vi "MotionProfileTest.vi"() -> ()   [LabVIEW 2018]
uses:
  <vilib>/Rock Robotics/WPI/ThirdParty/Phoenix-LabVIEW/Motor Controller/Controls/CTRE_Phoenix_MotorControl_TrajectoryPointTimeDur.ctl
  TypeDefs/MotionProfileGeneratorParams.ctl
panel:
  out "IntegralV":dbl
  out "NumPoints":i32
  out "Update Rate (Hz)":dbl
  in  "stop":bool
  out "Motion Profile":T1(graph)
  in  "Starting Position (units)":dbl
  in  "Acceleration Ramp Time (ms)":dbl=200.0
  in  "Trajectory Point Interval (ms)":T2=10 items=["TrajectoryDuration_0ms"=0, "TrajectoryDuration_5ms"=5, "TrajectoryDuration_10ms"=10, "TrajectoryDuration_20ms"=20, "TrajectoryDuration_30ms"=30, "TrajectoryDuration_40ms"=40, "TrajectoryDuration_50ms"=50, "TrajectoryDuration_100ms"=100]
  in  "Velocity Ramp Time (ms)":dbl=400.0
  in  "Maximum Travel Speed (units/s)":dbl=240.0
  in  "Travel Distance (units)":dbl=5.0
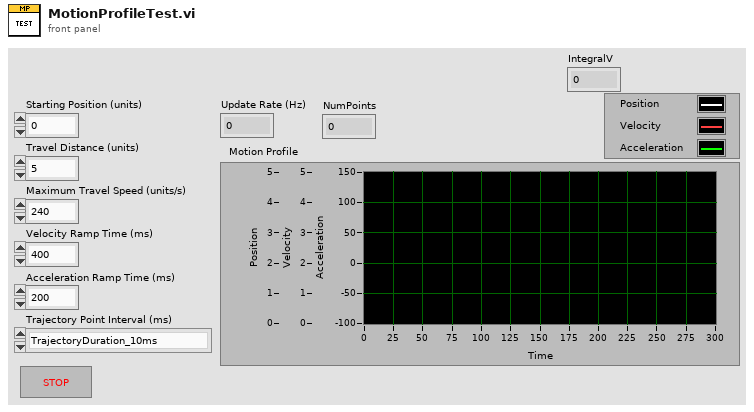
[diagram p1: front panel]
types:
  T1 = cluster{dbl, "Trajectory Point Interval (ms)":i32, dbl[][]}
  T2 = typedef "CTRE_Phoenix_MotorControl_TrajectoryPointTimeDur.ctl" = i32
  T3 = typedef "MotionProfileGeneratorParams.ctl" = cluster{"Trajectory Point Interval (ms)":T2, "Maximum Travel Speed (units/s)":dbl, "Velocity Ramp Time (ms)":dbl, "Acceleration Ramp Time (ms)":dbl}
  T4 = typedef "TrajectoryPoint.ctl" = cluster{"Position ":dbl, "Velocity ":dbl, "Time (ms)":T2, "Last Point":bool}
  T5 = cluster{dbl, "Trajectory Point Interval (ms)":T2, dbl[][]}
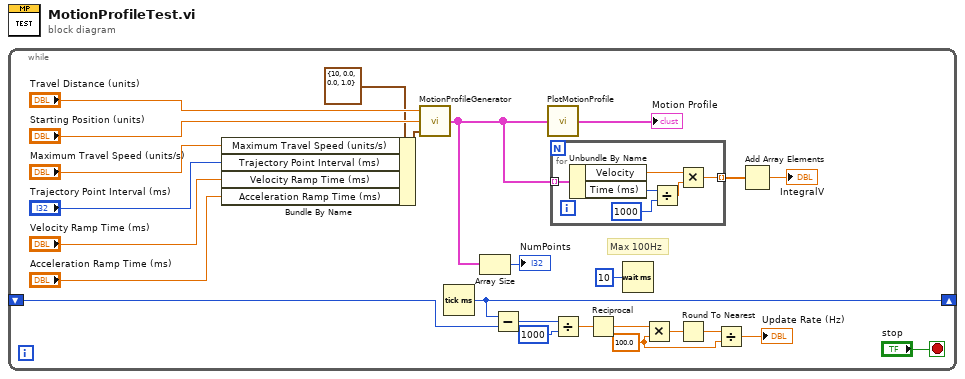
[diagram p0: block diagram]
diagram:
  n1 = while {
    shift-right: [w21] -> _
    shift-left: _ -> [w22]
    stop <- "stop" stop-if-true
    w14 = 100.0 ("y")
    # "Max 100Hz"
    n2 = Bundle By Name(cluster=T3 {"Trajectory Point Interval (ms)"=10, "Maximum Travel Speed (units/s)"=0.0, "Velocity Ramp Time (ms)"=0.0, "Acceleration Ramp Time (ms)"=1.0} ("MotionProfileGeneratorParameters"), "Maximum Travel Speed (units/s)"="Maximum Travel Speed (units/s)", "Trajectory Point Interval (ms)"="Trajectory Point Interval (ms)", "Velocity Ramp Time (ms)"="Velocity Ramp Time (ms)", "Acceleration Ramp Time (ms)"="Acceleration Ramp Time (ms)") -> (w9:T3)
    n3 = call "MotionProfileGenerator.vi"("MotionProfileGeneratorParameters"=w9, "Starting Position (units)"="Starting Position (units)", "Travel Distance (units)"="Travel Distance (units)") -> ("Trajectory Points"=w3:T4[])
    n4 = Tick Count (ms)() -> (millisecond timer value=w21:u32)
    n5 = Array Size(array=w3) -> (size(s)=→"NumPoints":i32)
    n6 = Subtract(x=w21, y=w22) -> (x-y=w20:u32)
    n7 = call "PlotMotionProfile.vi"("Trajectory Points"=w3) -> ("MotionProfileGraph"=→"Motion Profile":T5)
    n8 = for {
      tunnel: w3 -> [w31] mode=indexing
      tunnel: [w29] -> w2 mode=indexing
      n9 = Unbundle By Name(w31) -> ("Velocity"=w30:dbl, "Time (ms)"=w28:T2)
      n10 = Divide(x=w28, y=1000) -> (x/y=w27:dbl)
      n11 = Multiply(x=w30, y=w27) -> (x*y=w29:dbl)
    }
    n12 = Divide(x=w20, y=u32 1000) -> (x/y=w18:dbl)
    n13 = Reciprocal(x=w18) -> (1/x=w17:dbl)
    n14 = Wait (ms)(milliseconds to wait=u32 10) -> ()  [unwired: 1 out]
    n15 = Multiply(x=w17, y=w14) -> (x*y=w16:dbl)
    n16 = Round To Nearest(number=w16) -> (nearest integer value=w15:dbl)
    n17 = Divide(x=w15, y=w14) -> (x/y=→"Update Rate (Hz)":dbl)
    n18 = Add Array Elements(numeric array=w2) -> (sum=→"IntegralV":dbl)
  }
